vi "Change Activation Type.vi"(7 "Tab Selector":T2(ring), 8 "Ligasure - Tab":T6, 9 "Bipolar - Tab":T5, 10 "Mono2 - Tab":T4, 11 "Mono1 - Tab":T3) -> (0 "Ligasure - Tab Enum":T1, 1 "Bipolar - Tab Enum":T1, 2 "Mono2 - Tab Enum":T1, 3 "Mono1 - Tab Enum":T1)   [LabVIEW 2024]
uses:
  Controls/Tab Enums/Activation Type Enum.ctl
  Controls/Tab Enums/Ligasure - Tab.ctl
  Controls/Tab Enums/Bipolar - Tab.ctl
  Controls/Tab Enums/Mono2 - Tab.ctl
  Controls/Tab Enums/Mono1 - Tab.ctl
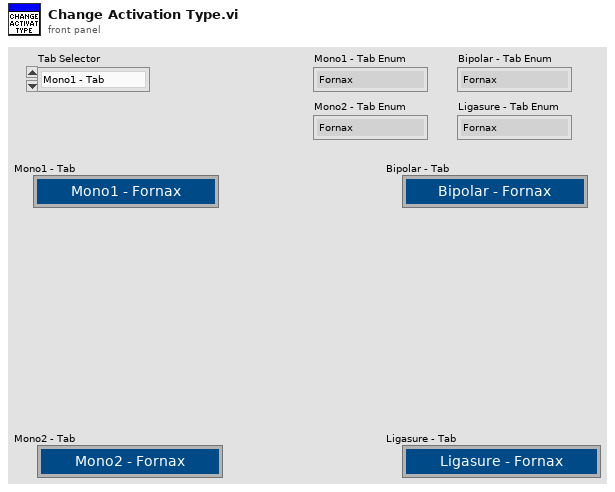
[diagram p1: front panel]
types:
  T1 = typedef "Activation Type Enum.ctl" = enum16{"Fornax", "Handswitch", "Footswitch", "Triverse", "Auto Bipolar"}
  T2 = enum16{"Mono1 - Tab", "Mono2 - Tab", "Bipolar - Tab", "Ligasure - Tab"}
  T3 = typedef "Mono1 - Tab.ctl" = enum32{"Mono1 - Fornax", "Mono1 - Handswitch", "Mono1 - Footswitch"}
  T4 = typedef "Mono2 - Tab.ctl" = enum32{"Mono2 - Fornax", "Mono2 - Handswitch", "Mono2 - Footswitch", "Mono2 - Triverse"}
  T5 = typedef "Bipolar - Tab.ctl" = enum32{"Bipolar - Fornax", "Bipolar - Handswitch", "Bipolar - Footswitch", "Auto Bipolar"}
  T6 = typedef "Ligasure - Tab.ctl" = enum32{"Ligasure - Fornax", "Ligasure - Handswitch", "Ligasure - Footswitch"}
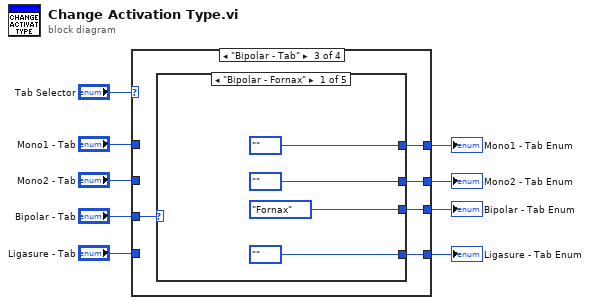
[diagram p0: block diagram]
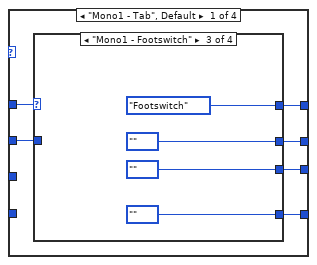
[diagram p2: hidden frame]
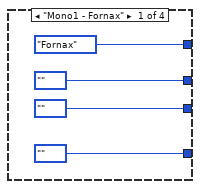
[diagram p3: hidden frame]
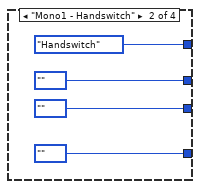
[diagram p4: hidden frame]
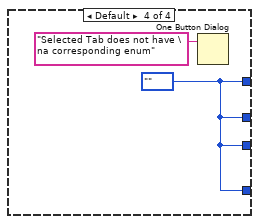
[diagram p5: hidden frame]
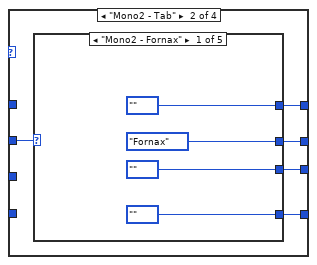
[diagram p6: hidden frame]
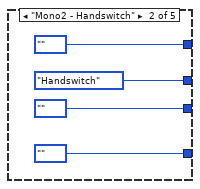
[diagram p7: hidden frame]
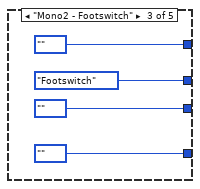
[diagram p8: hidden frame]
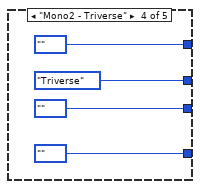
[diagram p9: hidden frame]
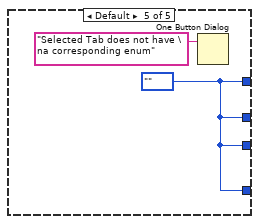
[diagram p10: hidden frame]
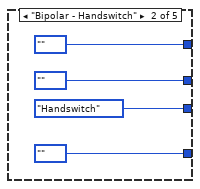
[diagram p11: hidden frame]
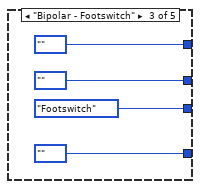
[diagram p12: hidden frame]
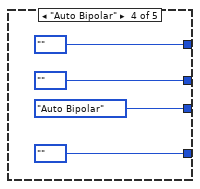
[diagram p13: hidden frame]
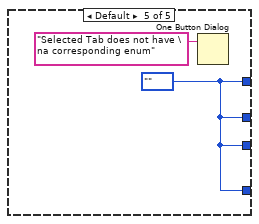
[diagram p14: hidden frame]
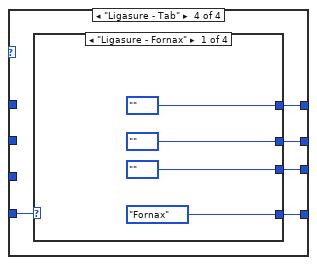
[diagram p15: hidden frame]
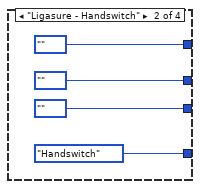
[diagram p16: hidden frame]
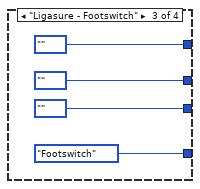
[diagram p17: hidden frame]
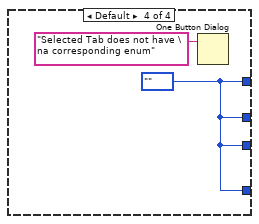
[diagram p18: hidden frame]
diagram:
  n1 = case shown="\"Bipolar - Tab\"" "Tab Selector" {
    tunnel: "Mono1 - Tab" -> [w15 _ _ _]
    tunnel: [w14 w34 w57 w80] -> w4
    tunnel: "Mono2 - Tab" -> [w13 w33 _ _]
    tunnel: [w12 w32 w56 w79] -> w3
    tunnel: "Bipolar - Tab" -> [_ _ w55 _]
    tunnel: [w11 w31 w54 w78] -> w2
    tunnel: "Ligasure - Tab" -> [_ _ _ w77]
    tunnel: [w10 w30 w53 w76] -> w1
    frame "Mono1 - Tab", Default {
      n2 = case shown="\"Mono1 - Footswitch\"" w15 {
        tunnel: [Activation_Type_Enum."Fornax" ("Activation Type Enum") Activation_Type_Enum."Handswitch" ("Activation Type Enum") Activation_Type_Enum."Footswitch" ("Activation Type Enum") w28] -> w14
        tunnel: w13 -> [_ _ _ _]
        tunnel: [enum16{""}."" enum16{""}."" enum16{""}."" w28] -> w12
        tunnel: [enum16{""}."" enum16{""}."" enum16{""}."" w28] -> w11
        tunnel: [enum16{""}."" enum16{""}."" enum16{""}."" w28] -> w10
        frame "Mono1 - Fornax" {
        }
        frame "Mono1 - Handswitch" {
        }
        frame "Mono1 - Footswitch" {
        }
        frame Default {
          w28 = enum16{""}.""
          n3 = One Button Dialog(message="Selected Tab does not have \na corresponding enum") -> ()  [unwired: 1 in, 1 out]
        }
      }
    }
    frame "Mono2 - Tab" {
      n4 = case shown="\"Mono2 - Fornax\"" w33 {
        tunnel: [enum16{""}."" enum16{""}."" enum16{""}."" enum16{""}."" w51] -> w34
        tunnel: [Activation_Type_Enum."Fornax" ("Activation Type Enum") Activation_Type_Enum."Handswitch" ("Activation Type Enum") Activation_Type_Enum."Footswitch" ("Activation Type Enum") Activation_Type_Enum."Triverse" ("Activation Type Enum") w51] -> w32
        tunnel: [enum16{""}."" enum16{""}."" enum16{""}."" enum16{""}."" w51] -> w31
        tunnel: [enum16{""}."" enum16{""}."" enum16{""}."" enum16{""}."" w51] -> w30
        frame "Mono2 - Fornax" {
        }
        frame "Mono2 - Handswitch" {
        }
        frame "Mono2 - Footswitch" {
        }
        frame "Mono2 - Triverse" {
        }
        frame Default {
          w51 = enum16{""}.""
          n5 = One Button Dialog(message="Selected Tab does not have \na corresponding enum") -> ()  [unwired: 1 in, 1 out]
        }
      }
    }
    frame "Bipolar - Tab" {
      n6 = case shown="\"Bipolar - Fornax\"" w55 {
        tunnel: [enum16{""}."" enum16{""}."" enum16{""}."" enum16{""}."" w74] -> w57
        tunnel: [enum16{""}."" enum16{""}."" enum16{""}."" enum16{""}."" w74] -> w56
        tunnel: [Activation_Type_Enum."Fornax" ("Activation Type Enum") Activation_Type_Enum."Handswitch" ("Activation Type Enum") Activation_Type_Enum."Footswitch" ("Activation Type Enum") Activation_Type_Enum."Auto Bipolar" ("Activation Type Enum") w74] -> w54
        tunnel: [enum16{""}."" enum16{""}."" enum16{""}."" enum16{""}."" w74] -> w53
        frame "Bipolar - Fornax" {
        }
        frame "Bipolar - Handswitch" {
        }
        frame "Bipolar - Footswitch" {
        }
        frame "Auto Bipolar" {
        }
        frame Default {
          w74 = enum16{""}.""
          n7 = One Button Dialog(message="Selected Tab does not have \na corresponding enum") -> ()  [unwired: 1 in, 1 out]
        }
      }
    }
    frame "Ligasure - Tab" {
      n8 = case shown="\"Ligasure - Fornax\"" w77 {
        tunnel: [enum16{""}."" enum16{""}."" enum16{""}."" w93] -> w80
        tunnel: [enum16{""}."" enum16{""}."" enum16{""}."" w93] -> w79
        tunnel: [enum16{""}."" enum16{""}."" enum16{""}."" w93] -> w78
        tunnel: [Activation_Type_Enum."Fornax" ("Activation Type Enum") Activation_Type_Enum."Handswitch" ("Activation Type Enum") Activation_Type_Enum."Footswitch" ("Activation Type Enum") w93] -> w76
        frame "Ligasure - Fornax" {
        }
        frame "Ligasure - Handswitch" {
        }
        frame "Ligasure - Footswitch" {
        }
        frame Default {
          w93 = enum16{""}.""
          n9 = One Button Dialog(message="Selected Tab does not have \na corresponding enum") -> ()  [unwired: 1 in, 1 out]
        }
      }
    }
  }
  "Mono1 - Tab Enum" <- w4
  "Mono2 - Tab Enum" <- w3
  "Bipolar - Tab Enum" <- w2
  "Ligasure - Tab Enum" <- w1
